vi "settings handler.vi"(7 "Operation":enum16{"Open", "Write", "Read", "Close"}(ring), 8 "error in (no error)":errorcluster, 9 "Paths write":T1, 11 "Write":T2={"COM"="", "baud rate"=115200, "data bits"=8, "parity"=enum."None", "stop bits"=10, "flow control"=enum."None", "delay"=50, "I/O channel"=""} {"stop bits" items=["1.0"=10, "1.5"=15, "2.0"=20]; "baud rate" max=921600; "data bits" max=16}) -> (0 "Error Out":errorcluster, 1 "Paths read":T1, 3 "Read":T2={"COM"="", "baud rate"=115200, "data bits"=8, "parity"=enum."None", "stop bits"=10, "flow control"=enum."None", "delay"=50, "I/O channel"=""} {"stop bits" items=["1.0"=10, "1.5"=15, "2.0"=20]; "baud rate" max=921600; "data bits" max=16})   [LabVIEW 2021]
uses:
  <vilib>/Utility/config.llb/Write Key (String).vi
  <vilib>/Utility/config.llb/Read Key (String).vi
  <vilib>/Utility/config.llb/Read Key (U32).vi
  <vilib>/Utility/config.llb/NI_LVConfig.lvlib
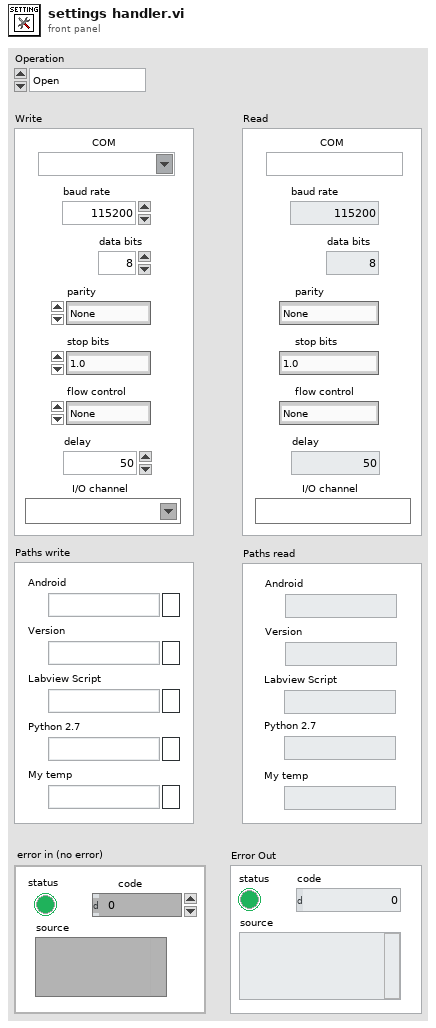
[diagram p1: front panel]
types:
  T1 = cluster{"Android":path, "Version":path, "Labview Script":path, "Python 2.7":path, "My temp":path}
  T2 = cluster{"COM":refnum<visa-resource-name>, "baud rate":u32, "data bits":u8, "parity":enum16{"None", "Odd", "Even", "Mark", "Space"}, "stop bits":u16, "flow control":enum16{"None", "XON/XOFF", "RTS/CTS", "DTR/DSR"}, "delay":u16, "I/O channel":refnum<k21>}
  T3 = typedef "NI_LVConfig.lvlib/Config Data RefNum.ctl" = refnum<k1>
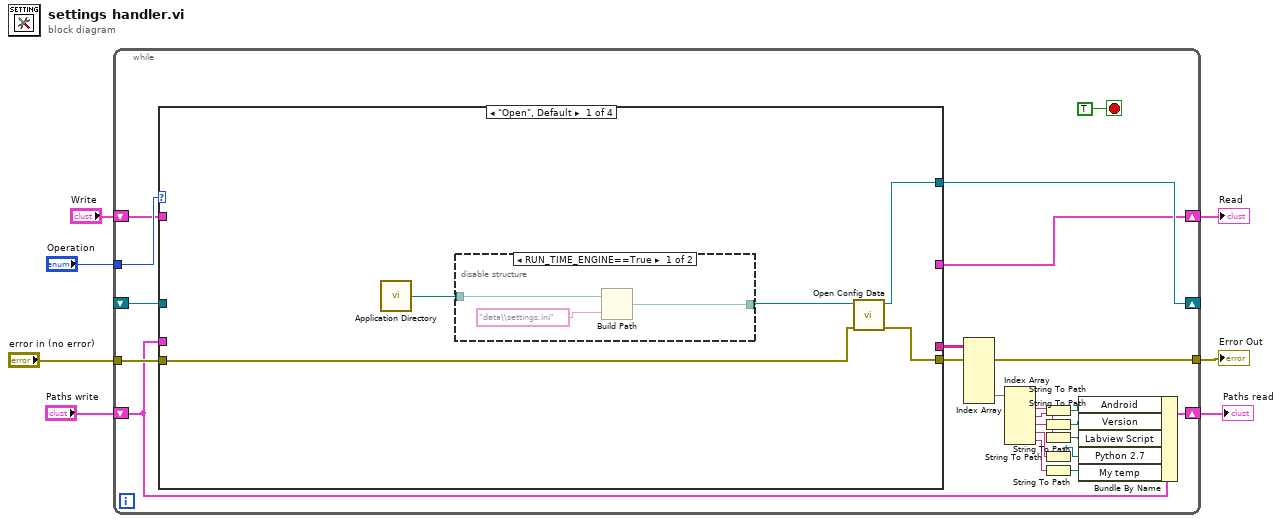
[diagram p0: block diagram]
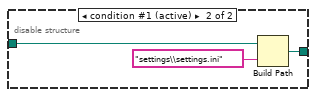
[diagram p2: hidden frame]
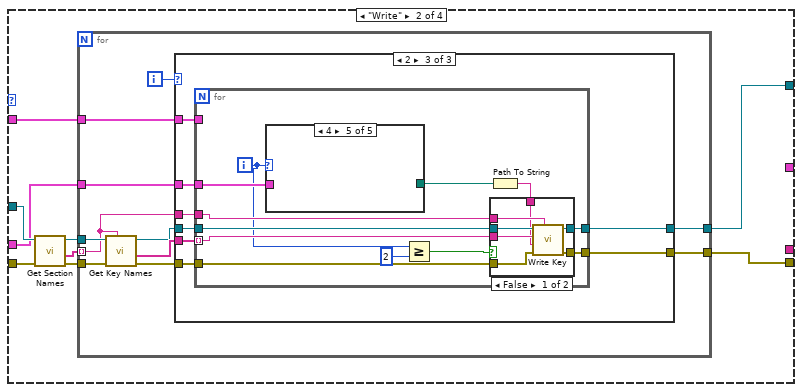
[diagram p3: hidden frame]
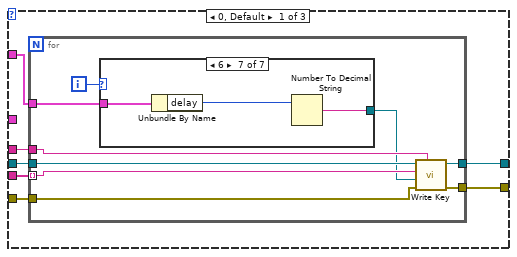
[diagram p4: hidden frame]
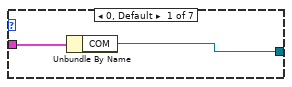
[diagram p5: hidden frame]
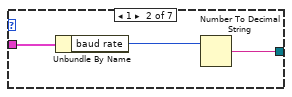
[diagram p6: hidden frame]
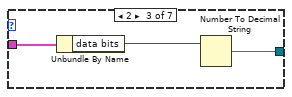
[diagram p7: hidden frame]
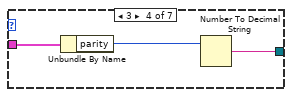
[diagram p8: hidden frame]
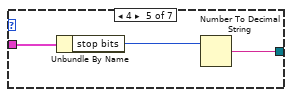
[diagram p9: hidden frame]
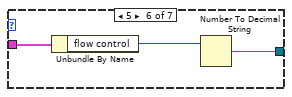
[diagram p10: hidden frame]
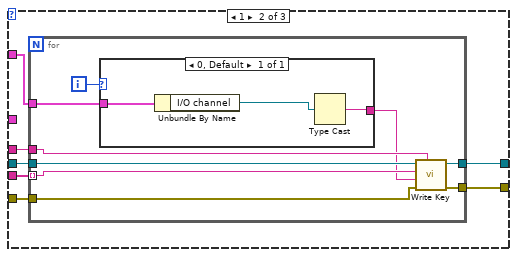
[diagram p11: hidden frame]
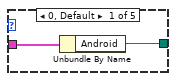
[diagram p13: hidden frame]
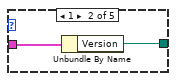
[diagram p14: hidden frame]
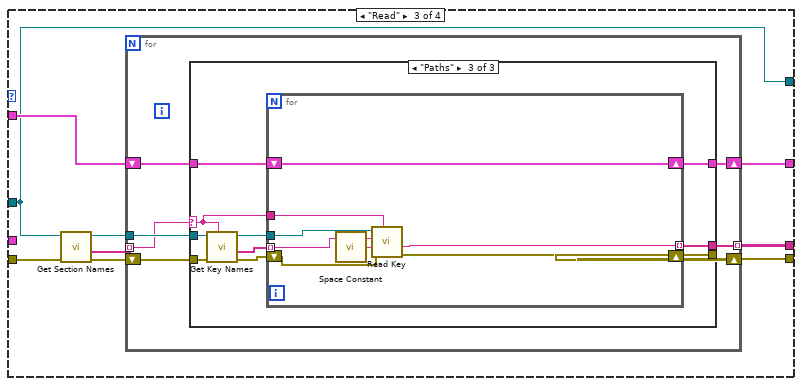
[diagram p17: hidden frame]
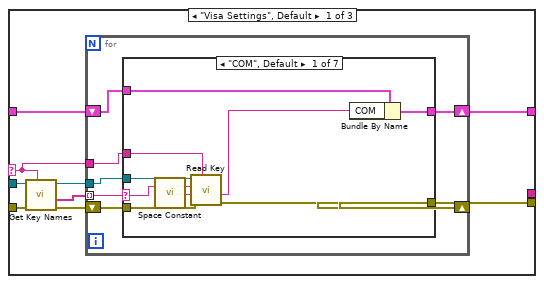
[diagram p18: hidden frame]
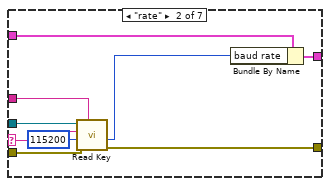
[diagram p19: hidden frame]
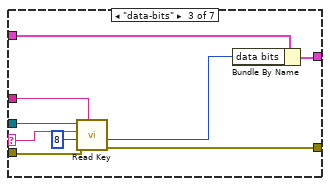
[diagram p20: hidden frame]
diagram:
  n1 = while {
    tunnel: "error in (no error)" -> [w29]
    tunnel: [w28] -> w6
    shift-right: [w27] -> _
    shift-left: _ -> [w25]
    shift-right: [w18] -> w3
    shift-left: "Write" -> [w23]
    tunnel: "Operation" -> [w24]
    shift-right: [w21] -> w1
    shift-left: "Paths write" -> [w22]
    stop <- TRUE stop-if-true
    n2 = case shown="\"Open\", Default" w24 {
      tunnel: w29 -> [w34 w46 w157 w289]
      tunnel: [w33 w42 w154 w288] -> w28
      tunnel: [w32 w43 w149 _] -> w27
      tunnel: w25 -> [_ w45 w149 w287]
      tunnel: w23 -> [_ w44 w152 _]
      tunnel: w22 -> [_ w41 _ _]
      tunnel: [_ _ w153 _] -> w18
      tunnel: [_ _ w151 _] -> w17
      frame "Open", Default {
        n3 = call <vilib>:"Application Directory.vi"() -> ("Application Directory"=w31:path)
        n4 = disable-structure shown="RUN_TIME_ENGINE==True" {
          disable-tunnel: [w36 w39] -> w30
          disable-tunnel: w31 -> [w35 w38]
          frame condition #0 {
            n5 = Build Path(base path=w35, name or relative path="data\\settings.ini") -> (appended path=w36:path)
          }
          frame condition #1 (active) {
            n6 = Build Path(base path=w38, name or relative path="settings\\settings.ini") -> (appended path=w39:path)
          }
        }
        n7 = call <vilib>:"Open Config Data.vi"("error in (no error)"=w34, "configuration file path"=w30) -> ("error out"=w33:errorcluster, "refnum"=w32:T3)  [unwired: 7 in, 1 out]
      }
      frame "Write" {
        n8 = call <vilib>:"Get Section Names.vi"("error in (no error)"=w46, "refnum"=w45) -> ("error out"=w47:errorcluster, "section names"=w49:string[], "refnum out"=w48:T3)  [unwired: 7 in]
        n9 = for {
          tunnel: w49 -> [w58] mode=indexing
          tunnel: w48 -> [w60]
          tunnel: w47 -> [w59]
          tunnel: [w54] -> w43
          tunnel: [w53] -> w42
          tunnel: w44 -> [w52]
          tunnel: w41 -> [w50]
          i -> [w51]
          n10 = call <vilib>:"Get Key Names.vi"("section"=w58, "error in (no error)"=w59, "refnum"=w60) -> ("error out"=w55:errorcluster, "key names"=w57:string[], "refnum out"=w56:T3)  [unwired: 5 in, 1 out]
          n11 = case shown="2" w51 {
            tunnel: w58 -> [w67 w103 w123]
            tunnel: w57 -> [w66 w102 w122]
            tunnel: w56 -> [w65 w101 w121]
            tunnel: w55 -> [w64 w100 w120]
            tunnel: [w63 w99 w119] -> w54
            tunnel: [w62 w98 w118] -> w53
            tunnel: w52 -> [w61 w97 w117]
            tunnel: w50 -> [_ _ w116]
            frame 0, Default {
              n12 = for {
                tunnel: w67 -> [w76]
                tunnel: w66 -> [w75] mode=indexing
                tunnel: w65 -> [w74]
                tunnel: w64 -> [w73]
                tunnel: [w72] -> w63
                tunnel: [w71] -> w62
                tunnel: w61 -> [w69]
                i -> [w70]
                n13 = case shown="6" w70 {
                  tunnel: w69 -> [w78 w81 w84 w87 w90 w93 w96]
                  tunnel: [w77 w79 w82 w85 w88 w91 w94] -> w68
                  frame 0, Default {
                    n14 = Unbundle By Name(w78) -> ("COM"=w77:refnum<visa-resource-name>)
                  }
                  frame 1 {
                    n15 = Unbundle By Name(w81) -> ("baud rate"=w80:u32)
                    n16 = Number To Decimal String(number=w80) -> (decimal integer string=w79:string)  [unwired: 1 in]
                  }
                  frame 2 {
                    n17 = Unbundle By Name(w84) -> ("data bits"=w83:u8)
                    n18 = Number To Decimal String(number=w83) -> (decimal integer string=w82:string)  [unwired: 1 in]
                  }
                  frame 3 {
                    n19 = Unbundle By Name(w87) -> ("parity"=w86:enum16{"None", "Odd", "Even", "Mark", "Space"})
                    n20 = Number To Decimal String(number=w86) -> (decimal integer string=w85:string)  [unwired: 1 in]
                  }
                  frame 4 {
                    n21 = Unbundle By Name(w90) -> ("stop bits"=w89:u16)
                    n22 = Number To Decimal String(number=w89) -> (decimal integer string=w88:string)  [unwired: 1 in]
                  }
                  frame 5 {
                    n23 = Unbundle By Name(w93) -> ("flow control"=w92:enum16{"None", "XON/XOFF", "RTS/CTS", "DTR/DSR"})
                    n24 = Number To Decimal String(number=w92) -> (decimal integer string=w91:string)  [unwired: 1 in]
                  }
                  frame 6 {
                    n25 = Unbundle By Name(w96) -> ("delay"=w95:u16)
                    n26 = Number To Decimal String(number=w95) -> (decimal integer string=w94:string)  [unwired: 1 in]
                  }
                }
                n27 = call-poly <vilib>:"Write Key.vi"("section"=w76, "error in (no error)"=w73, "value"=w68, "key"=w75, "refnum"=w74) -> ("error out"=w71:errorcluster, "refnum out"=w72:T3)  [unwired: 4 in, 1 out]
              }
            }
            frame 1 {
              n28 = for {
                tunnel: w103 -> [w112]
                tunnel: w102 -> [w111] mode=indexing
                tunnel: w101 -> [w110]
                tunnel: w100 -> [w109]
                tunnel: [w108] -> w99
                tunnel: [w107] -> w98
                tunnel: w97 -> [w105]
                i -> [w106]
                n29 = case shown="0, Default" w106 {
                  tunnel: w105 -> [w115]
                  tunnel: [w114] -> w104
                  frame 0, Default {
                    n30 = Unbundle By Name(w115) -> ("I/O channel"=w113:refnum<k21>)
                    n31 = Type Cast(x=w113) -> (*(type *) &x=w114:string)  [unwired: 1 in]
                  }
                }
                n32 = call-poly <vilib>:"Write Key.vi"("section"=w112, "error in (no error)"=w109, "value"=w104, "key"=w111, "refnum"=w110) -> ("error out"=w107:errorcluster, "refnum out"=w108:T3)  [unwired: 4 in, 1 out]
              }
            }
            frame 2 {
              n33 = for {
                tunnel: w123 -> [w135]
                tunnel: w122 -> [w134] mode=indexing
                tunnel: w121 -> [w133]
                tunnel: w120 -> [w132]
                tunnel: [w131] -> w119
                tunnel: [w130] -> w118
                tunnel: w117 -> [_]
                tunnel: w116 -> [w129]
                i -> [w126]
                n34 = case shown="4" w126 {
                  tunnel: w129 -> [w145 w148 _ _ _]
                  tunnel: [w146 w147 _ _ _] -> w128
                  frame 0, Default {
                    n35 = Unbundle By Name(w145) -> ("Android"=w146:path)
                  }
                  frame 1 {
                    n36 = Unbundle By Name(w148) -> ("Version"=w147:path)
                  }
                  frame 2 {
                  }
                  frame 3 {
                  }
                  frame 4 {
                  }
                }
                n37 = Greater Or Equal?(x=w126, y=2) -> (x >= y?=w124:bool)
                n38 = Path To String(path=w128) -> (string=w127:string)
                n39 = case shown="False" w124 {
                  tunnel: w135 -> [w142 _]
                  tunnel: w134 -> [w141 _]
                  tunnel: w133 -> [w140 w144]
                  tunnel: w132 -> [w139 w143]
                  tunnel: [w138 w144] -> w131
                  tunnel: [w137 w143] -> w130
                  tunnel: w127 -> [w136 _]
                  frame False {
                    n40 = call-poly <vilib>:"Write Key.vi"("section"=w142, "error in (no error)"=w139, "value"=w136, "key"=w141, "refnum"=w140) -> ("error out"=w137:errorcluster, "refnum out"=w138:T3)  [unwired: 4 in, 1 out]
                  }
                  frame True {
                  }
                }
              }
            }
          }
        }
      }
      frame "Read" {
        n41 = call <vilib>:"Get Section Names.vi"("error in (no error)"=w157, "refnum"=w149) -> ("error out"=w155:errorcluster, "section names"=w156:string[], "refnum out"=w150:T3)  [unwired: 7 in]
        n42 = for {
          tunnel: w156 -> [w162] mode=indexing
          tunnel: w150 -> [w164]
          shift-right: [w161] -> w154
          shift-left: w155 -> [w163]
          shift-right: [w160] -> w153
          shift-left: w152 -> [w159]
          tunnel: [w158] -> w151 mode=indexing
          n43 = case shown="\"Paths\"" w162 {
            selector: w162 -> [w168 w247 w273]
            tunnel: w164 -> [w173 w252 w278]
            tunnel: w163 -> [w172 w251 w277]
            tunnel: [w167 w246 w272] -> w161
            tunnel: [w166 w244 w270] -> w160
            tunnel: w159 -> [w165 w245 w271]
            tunnel: [_ _ w269] -> w158
            frame "Visa Settings", Default {
              n44 = call <vilib>:"Get Key Names.vi"("section"=w168, "error in (no error)"=w172, "refnum"=w173) -> ("error out"=w169:errorcluster, "key names"=w171:string[], "refnum out"=w170:T3)  [unwired: 5 in, 1 out]
              n45 = for {
                tunnel: w168 -> [w179]
                tunnel: w171 -> [w180] mode=indexing
                tunnel: w170 -> [w178]
                shift-right: [w176] -> w167
                shift-left: w169 -> [w177]
                shift-right: [w175] -> w166
                shift-left: w165 -> [w174]
                n46 = case shown="\"COM\", Default" w180 {
                  selector: w180 -> [w188 w197 w206 w215 w224 w233 w242]
                  tunnel: w179 -> [w189 w198 w207 w216 w225 w234 w243]
                  tunnel: w178 -> [w187 w196 w205 w208 w223 w232 w241]
                  tunnel: w177 -> [w186 w195 w204 w213 w221 w231 w240]
                  tunnel: [w184 w193 w202 w212 w220 w229 w238] -> w176
                  tunnel: w174 -> [w182 w192 w200 w210 w218 w227 w236]
                  tunnel: [w183 w191 w201 w211 w219 w228 w237] -> w175
                  frame "COM", Default {
                    n47 = call <vilib>:"Space Constant.vi"() -> ("String"=w185:string)
                    n48 = call-poly <vilib>:"Read Key.vi"("section"=w189, "error in (no error)"=w186, "default value"=w185, "key"=w188, "refnum"=w187) -> ("error out"=w184:errorcluster, "value"=w181:string)  [unwired: 3 in, 2 out]
                    n49 = Bundle By Name(cluster=w182, "COM"=w181) -> (w183:T2)
                  }
                  frame "rate" {
                    n50 = call-poly <vilib>:"Read Key.vi"("section"=w198, "error in (no error)"=w195, "default value"=u32 115200, "key"=w197, "refnum"=w196) -> ("error out"=w193:errorcluster, "value"=w190:u32)  [unwired: 3 in, 2 out]
                    n51 = Bundle By Name(cluster=w192, "baud rate"=w190) -> (w191:T2)
                  }
                  frame "data-bits" {
                    n52 = call-poly <vilib>:"Read Key.vi"("section"=w207, "error in (no error)"=w204, "default value"=u32 8, "key"=w206, "refnum"=w205) -> ("error out"=w202:errorcluster, "value"=w199:u32)  [unwired: 3 in, 2 out]
                    n53 = Bundle By Name(cluster=w200, "data bits"=w199) -> (w201:T2)
                  }
                  frame "parity" {
                    n54 = call-poly <vilib>:"Read Key.vi"("section"=w216, "error in (no error)"=w213, "default value"=u32 0, "key"=w215, "refnum"=w208) -> ("error out"=w212:errorcluster, "value"=w209:u32)  [unwired: 3 in, 2 out]
                    n55 = Bundle By Name(cluster=w210, "parity"=w209) -> (w211:T2)
                  }
                  frame "stop-bits" {
                    n56 = call-poly <vilib>:"Read Key.vi"("section"=w225, "error in (no error)"=w221, "default value"=u32 10, "key"=w224, "refnum"=w223) -> ("error out"=w220:errorcluster, "value"=w217:u32)  [unwired: 3 in, 2 out]
                    n57 = Bundle By Name(cluster=w218, "stop bits"=w217) -> (w219:T2)
                  }
                  frame "flow" {
                    n58 = call-poly <vilib>:"Read Key.vi"("section"=w234, "error in (no error)"=w231, "default value"=u32 0, "key"=w233, "refnum"=w232) -> ("error out"=w229:errorcluster, "value"=w226:u32)  [unwired: 3 in, 2 out]
                    n59 = Bundle By Name(cluster=w227, "flow control"=w226) -> (w228:T2)
                  }
                  frame "delay" {
                    n60 = call-poly <vilib>:"Read Key.vi"("section"=w243, "error in (no error)"=w240, "default value"=u32 50, "key"=w242, "refnum"=w241) -> ("error out"=w238:errorcluster, "value"=w235:u32)  [unwired: 3 in, 2 out]
                    n61 = Bundle By Name(cluster=w236, "delay"=w235) -> (w237:T2)
                  }
                }
              }
            }
            frame "IO channels" {
              n62 = call <vilib>:"Get Key Names.vi"("section"=w247, "error in (no error)"=w251, "refnum"=w252) -> ("error out"=w248:errorcluster, "key names"=w250:string[], "refnum out"=w249:T3)  [unwired: 5 in, 1 out]
              n63 = for {
                tunnel: w247 -> [w258]
                tunnel: w250 -> [w259] mode=indexing
                tunnel: w249 -> [w257]
                shift-right: [w255] -> w246
                shift-left: w248 -> [w256]
                shift-right: [w253] -> w244
                shift-left: w245 -> [w254]
                n64 = case shown="\"channel\", Default" w259 {
                  selector: w259 -> [w267]
                  tunnel: w258 -> [w268]
                  tunnel: w257 -> [w266]
                  tunnel: w256 -> [w264]
                  tunnel: [w263] -> w255
                  tunnel: [w262] -> w253
                  tunnel: w254 -> [w261]
                  frame "channel", Default {
                    n65 = call <vilib>:"Space Constant.vi"() -> ("String"=w265:string)
                    n66 = call-poly <vilib>:"Read Key.vi"("section"=w268, "error in (no error)"=w264, "default value"=w265, "key"=w267, "refnum"=w266) -> ("error out"=w263:errorcluster, "value"=w260:string)  [unwired: 3 in, 2 out]
                    n67 = Bundle By Name(cluster=w261, "I/O channel"=w260) -> (w262:T2)
                  }
                }
              }
            }
            frame "Paths" {
              n68 = call <vilib>:"Get Key Names.vi"("section"=w273, "error in (no error)"=w277, "refnum"=w278) -> ("error out"=w274:errorcluster, "key names"=w276:string[], "refnum out"=w275:T3)  [unwired: 5 in, 1 out]
              n69 = for {
                tunnel: w273 -> [w285]
                tunnel: w276 -> [w286] mode=indexing
                tunnel: w275 -> [w284]
                shift-right: [w282] -> w272
                shift-left: w274 -> [w283]
                shift-right: [w280] -> w270
                shift-left: w271 -> [w280]
                tunnel: [w279] -> w269 mode=indexing
                n70 = call <vilib>:"Space Constant.vi"() -> ("String"=w281:string)
                n71 = call-poly <vilib>:"Read Key.vi"("section"=w285, "error in (no error)"=w283, "default value"=w281, "key"=w286, "refnum"=w284) -> ("error out"=w282:errorcluster, "value"=w279:string)  [unwired: 3 in, 2 out]
              }
            }
          }
        }
      }
      frame "Close" {
        n72 = call <vilib>:"Close Config Data.vi"("error in (no error)"=w289, "refnum"=w287) -> ("error out"=w288:errorcluster)  [unwired: 8 in, 1 out]
      }
    }
    n73 = Index Array(array=w17) -> (element #3=w16:string[])  [unwired: 6 in, 2 out]
    n74 = Index Array(array=w16) -> (element #1=w14:string, element #2=w15:string, element #3=w12:string, element #4=w11:string, element #5=w10:string)  [unwired: 5 in]
    n75 = String To Path(string=w14) -> (path=w20:path)
    n76 = String To Path(string=w15) -> (path=w19:path)
    n77 = String To Path(string=w12) -> (path=w13:path)
    n78 = String To Path(string=w11) -> (path=w9:path)
    n79 = String To Path(string=w10) -> (path=w8:path)
    n80 = Bundle By Name(cluster=w22, "Android"=w20, "Version"=w19, "Labview Script"=w13, "Python 2.7"=w9, "My temp"=w8) -> (w21:T1)
  }
  "Error Out" <- w6
  "Read" <- w3
  "Paths read" <- w1
